vi "MGCC_Version2_MGCC_FntStaMach_Visualization_OpalRT_HTBtwoBatt.vi"() -> ()   [LabVIEW 2016]
doc: "-----------------------------------------------------------------------------------------------------------------------\nCopyright <2019> <The University of Tennessee at Knoxville and the University of Tennessee Research Foundation>\nThis software is released under BSD-3 \nhttps://opensource.org/licenses/BSD-3-Clause \nAdditional license options available at https://utrf.tennessee.edu/industry/sample-agreements/\n-----------------------------------------------------------------------------------------------------------------------"
uses:
  Islanded Control/MGCC_IsdCon_global1.vi
  Resynchronization/MGCC_Resync_global.vi
  Model Management/Global_MdlMgmt.vi
  Communication/Global communication output.vi
  MGCC_FntStaMach_PV_Mode.vi
  PV Forecasting/Sub-VIs/f_MGCC_PVFcst_ActualPV.vi
  Communication/Global communication.vi
  Energy Management/Sub-VIs/f_MGCC_EnergyMgmt_CostSavings.vi
  Energy Management/Sub-VIs/Battery Dispatch.vi
  MGCC_FntStaMach_gobal.vi
  Abnormal Fault State Control/Sub_VIs/Fault_Abnormal_state.vi
  PV Forecasting/Lib/MGCC_PVFcst_dataIO.lvlib
  Energy Management/Lib/MGCC_EnergyMgmt_dataIO.lvlib
panel:
  out "Working state":string
  out "Red":bool
  out "Orange":bool
  out "Yellow":bool
  out "Green":bool
  out "MG Error State":errorcluster
  out "Battery Dispatch GC":dbl[](graph)
  out "Savings":dbl
  out "Communication":bool
  out "PV Forecast":dynamicdata(graph)
  out "APF 8":dbl format="%#.4f"
  out "APF 7":dbl format="%#.4f"
  out "APF 6":dbl format="%#.4f"
  out "APF 5":dbl format="%#.4f"
  out "APF 4":dbl format="%#.4f"
  out "APF 3":dbl format="%#.4f"
  out "APF 2":dbl format="%#.4f"
  out "APF 1":dbl format="%#.4f"
  out "?":bool
  out "?":bool
  out "?":bool
  in  "Load Mode":bool
  in  "?":dbl(slide) scale=0.0..2.0
  in  "PV Mode":bool
  out "Communication":bool
  out "Active power control":bool
  out "Reactive power control":bool
  out "Output":dbl format="%#_4f"
  out "Communication":bool
  out "Resynchronization":bool
  out "Active power control":bool
  out "Reactive power control":bool
  out "SOC 3":dbl format="%#_4f"
  out "Output":dbl format="%#_4f"
  out "Communication":bool
  out "Resynchronization":bool
  out "Active power control":bool
  out "Reactive power control":bool
  out "SOC":dbl format="%#_4f"
  out "Output":dbl format="%#_4f"
  out "I 8":dbl format="%#.4f"
  out "I 7":dbl format="%#.4f"
  out "I 6":dbl format="%#.4f"
  out "I 5":dbl format="%#.4f"
  out "I 4":dbl format="%#.4f"
  out "I 3":dbl format="%#.4f"
  out "I 2":dbl format="%#.4f"
  out "I 1":dbl format="%#.4f"
  out "Current State":string
  out "Model Mgmt.":bool
  out "PV Forecasting":bool
  out "Load Forecasting":bool
  out "PQ Balance":bool
  out "Black Start":bool
  out "Data Logging":bool
  out "State Estimation":bool
  out "Energy Mgmt.":bool
  out "L6":cluster{dbl[], dbl[]}(graph)
  out "L7":cluster{dbl[], dbl[]}(graph)
  out "L8":cluster{dbl[], dbl[]}(graph)
  out "B10":cluster{dbl[], dbl[]}(graph)
  out "PV":cluster{dbl[], dbl[]}(graph)
  out "L11":cluster{dbl[], dbl[]}(graph)
  out "L5":cluster{dbl[], dbl[]}(graph)
  out "G4":cluster{dbl[], dbl[]}(graph)
  out "B12":cluster{dbl[], dbl[]}(graph)
  out "L3":cluster{dbl[], dbl[]}(graph)
  out "L2":cluster{dbl[], dbl[]}(graph)
  out "G1":cluster{dbl[], dbl[]}(graph)
  in  "Stop":bool
  in  "RESET":bool
  in  "G2":bool
  in  "G1":bool
  in  "Ready for STD":bool
  in  "Recon cmd":bool
  in  "BKS cmd":bool
  in  "island cmd":bool
  out "Sources Power":T1(graph)
  in  "Power Tabs":T2(tab)
  out "Loads Power 2":dbl(graph)
  out "Loads Power 3":dbl(graph)
  out "Loads Power 5":dbl(graph)
  out "Loads Power 6":dbl(graph)
  out "Loads Power 7":dbl(graph)
  out "Loads Power 8":dbl(graph)
  out "Loads Power 11":dbl(graph)
  in  "Voltage Tabs":T2(tab)
  out "Voltage 2":dbl(graph)
  out "Voltage 3":dbl(graph)
  out "Voltage 5":dbl(graph)
  out "Voltage 6":dbl(graph)
  out "Voltage 7":dbl(graph)
  out "Voltage 8":dbl(graph)
  out "Voltage 11":dbl(graph)
  out "L6":bool
  out "L7":bool
  out "L8":bool
  out "B1":bool
  out "Bess1 Slider":dbl(slide) scale=0.0..1.0
  out "PV":bool
  out "L11":bool
  out "W9":bool
  out "I6":bool
  out "W5":bool
  out "I7":bool
  out "W6":bool
  out "I8":bool
  out "W7":bool
  out "I5":bool
  out "I4":bool
  out "W4":bool
  out "W3":bool
  out "I3":bool
  out "W8":bool
  out "I2":bool
  out "W2":bool
  out "I1":bool
  out "W1":bool
  out "L5":bool
  out "G4":bool
  out "B12":bool
  out "Bess2 Slider":dbl(slide) scale=0.0..1.0
  out "L3":bool
  out "L2":bool
  out "G1":bool
  # "Controller for Microgrid with Dynamic Boundary"
  # "Central Controller"
  # "BESS 12 Local Controller"
  # "BESS12"
  # "G4"
  # "L5"
  # "G1"
  # "L2"
  # "L3"
  # "Load profile \ncontrol"
  # "-Profile"
  # "-Manual"
  # "BESS10"
  # "L8"
  # "L6"
  # "PV9"
  # "L11"
  # "L7"
  # "PV9 Local Controller"
  # "BESS 10 Local Controller"
  # "-Profile"
  # "-Manual"
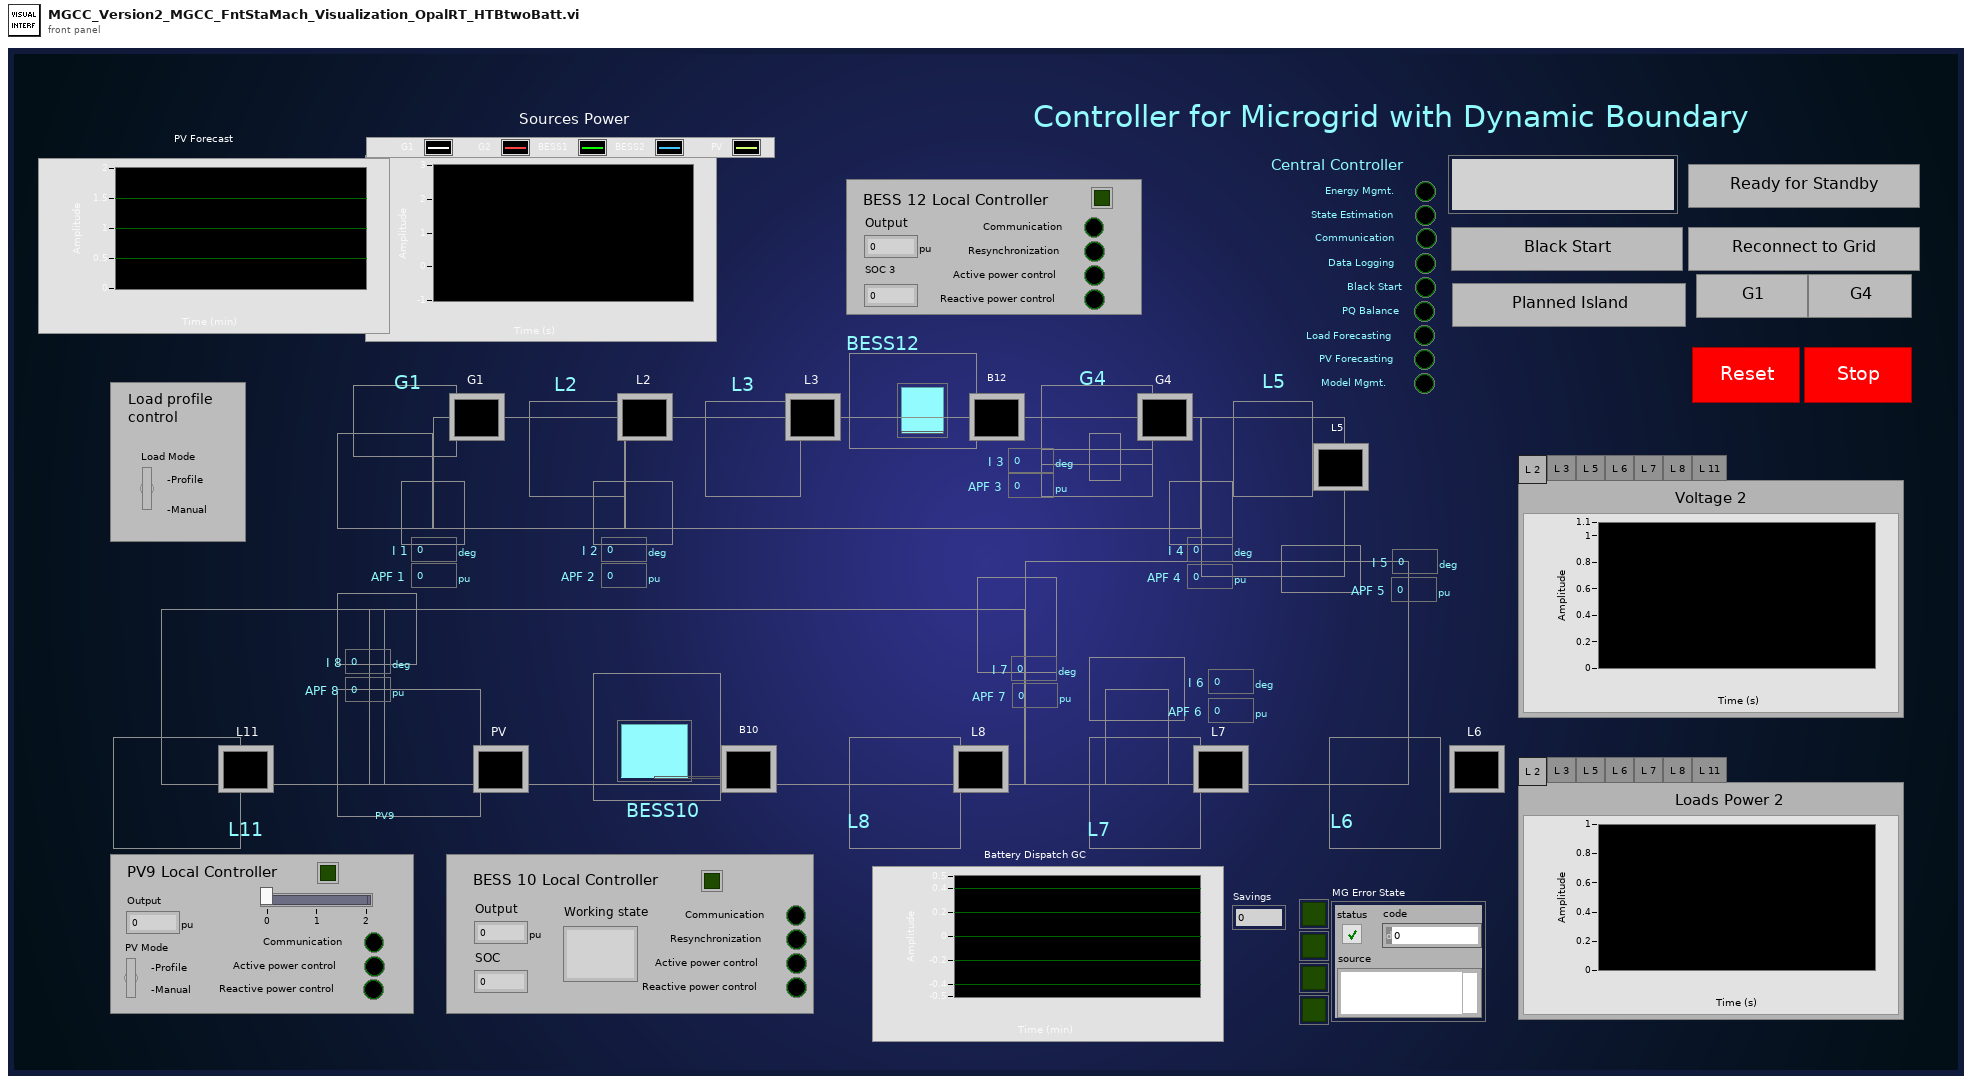
[diagram p1: front panel]
types:
  T1 = cluster{"Double":dbl, "Double":dbl, "Double":dbl, "Double":dbl, "Double":dbl}
  T2 = enum32{"L 2", "L 3", "L 5", "L 6", "L 7", "L 8", "L 11"}
  T3 = cluster{"Numeric":dbl, "Numeric":dbl, "Numeric":dbl, "Numeric":dbl}
  T4 = cluster{"Numeric":dbl, dbl, "Numeric":dbl, "Numeric":dbl, "Numeric":dbl}
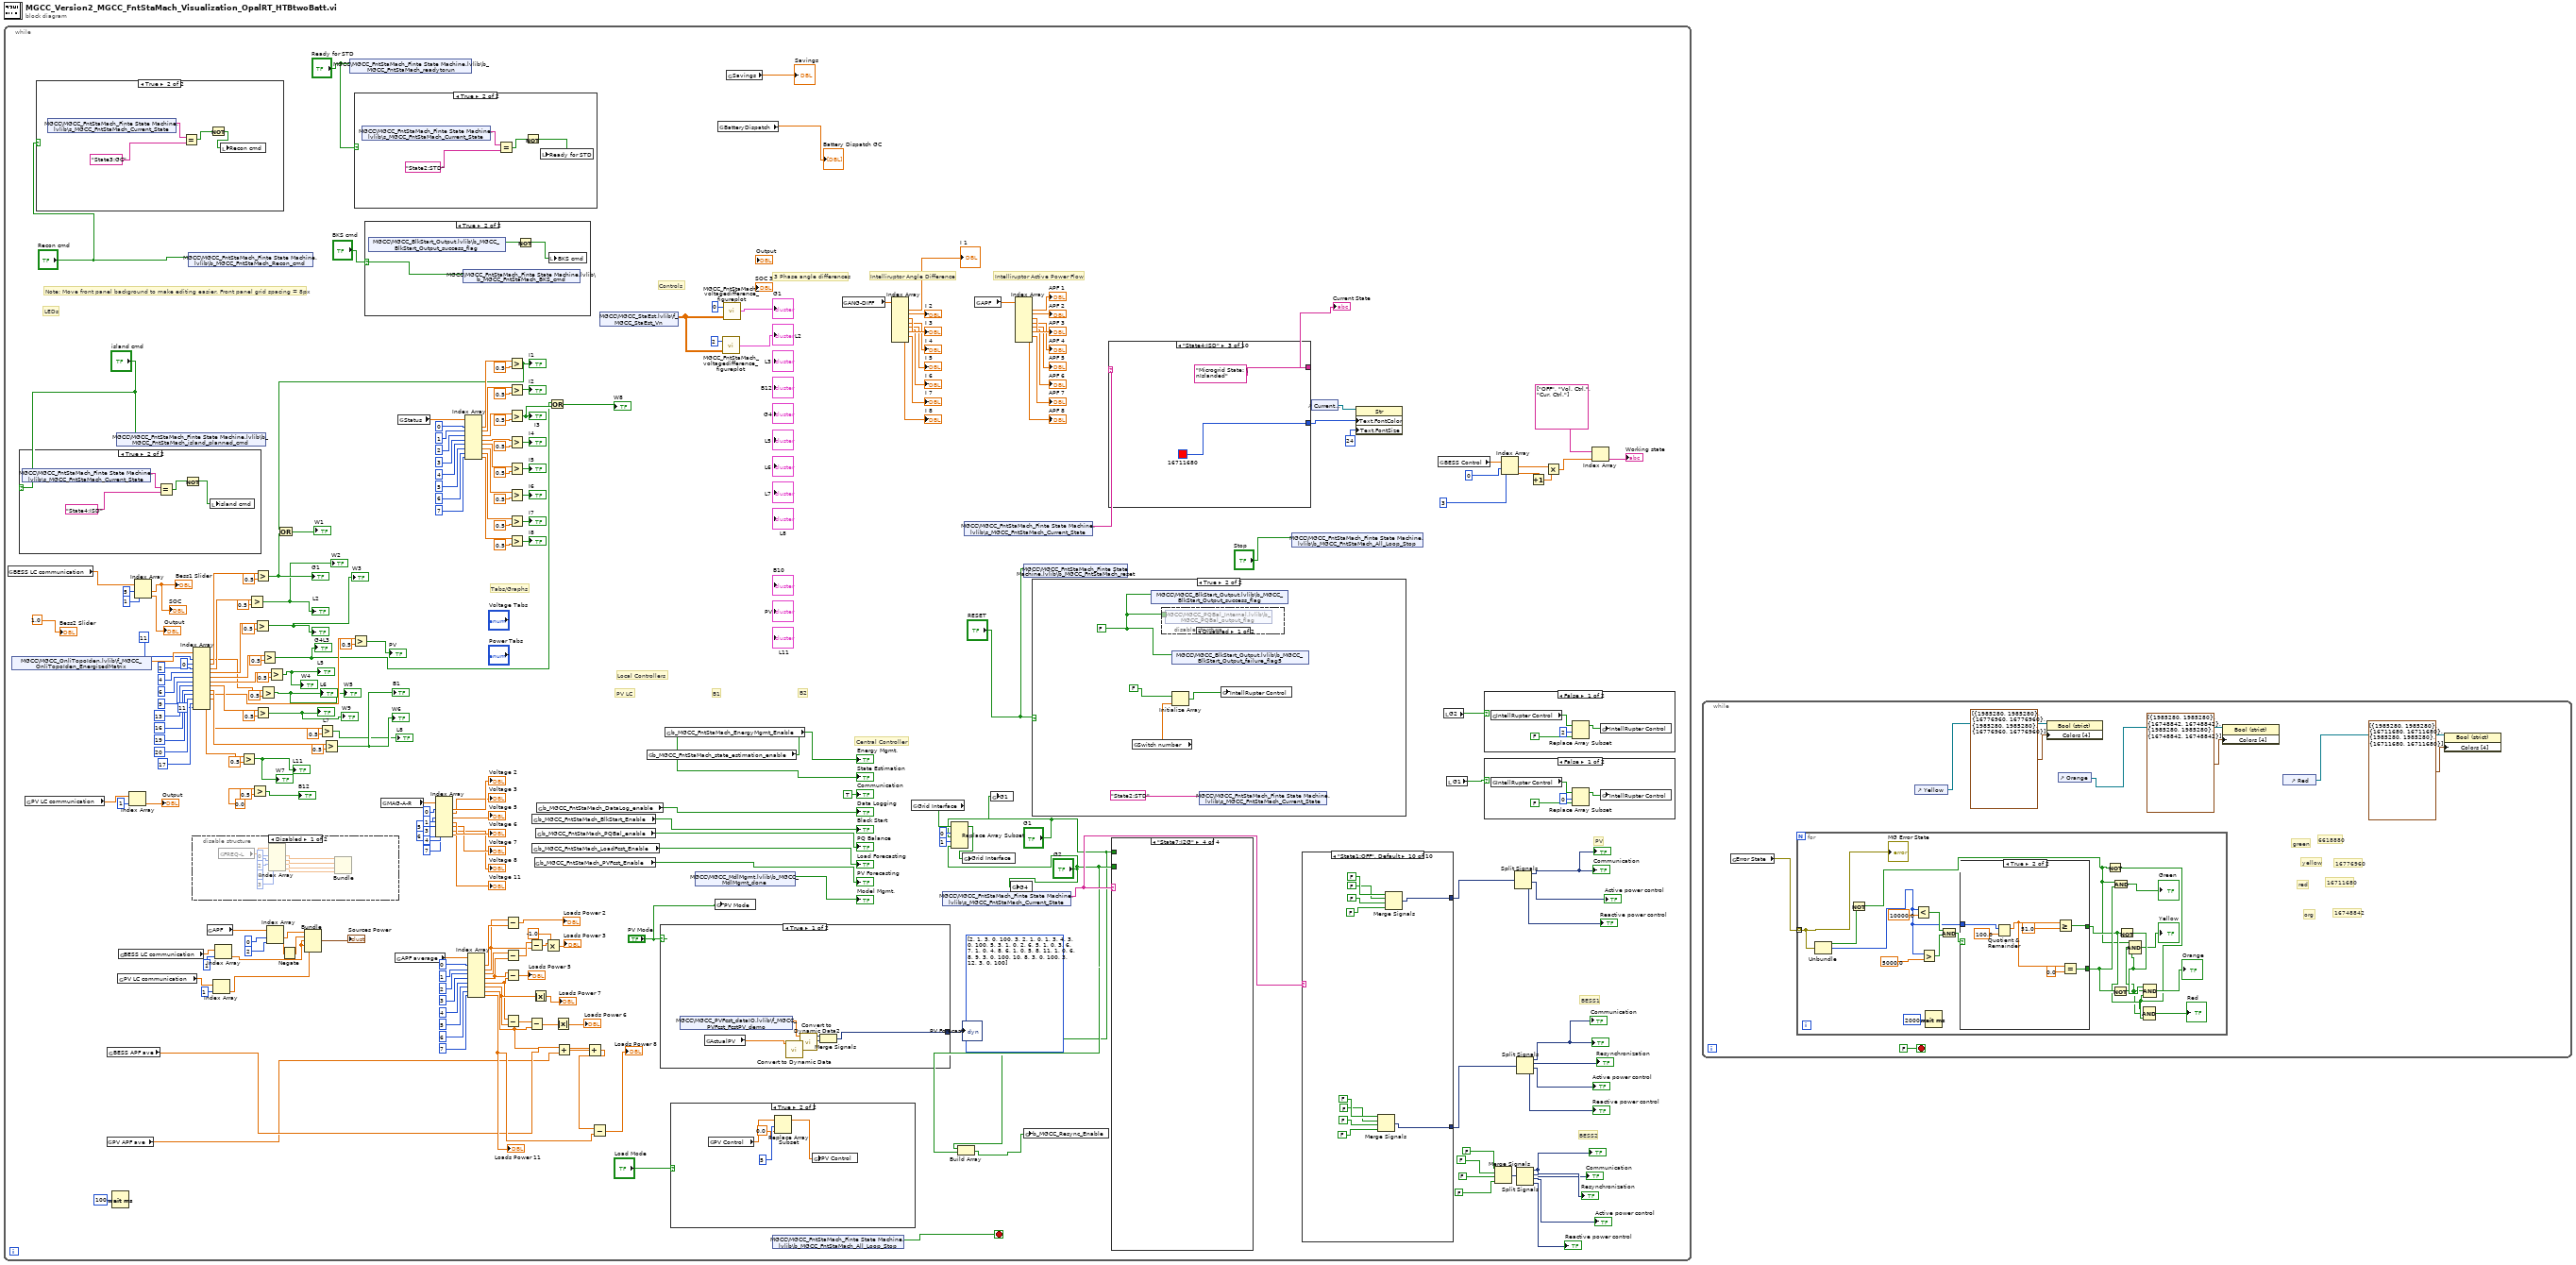
[diagram p0: block diagram]
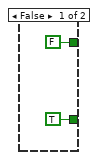
[diagram p2: hidden frame]
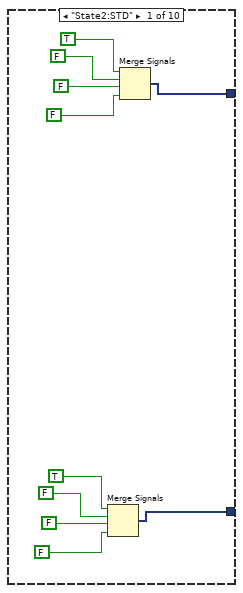
[diagram p8: hidden frame]
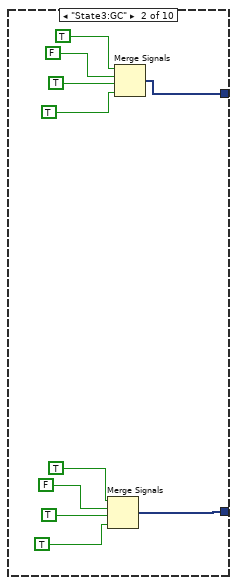
[diagram p9: hidden frame]
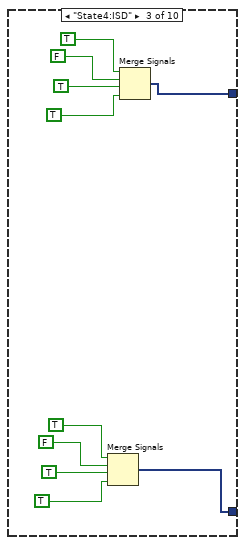
[diagram p10: hidden frame]
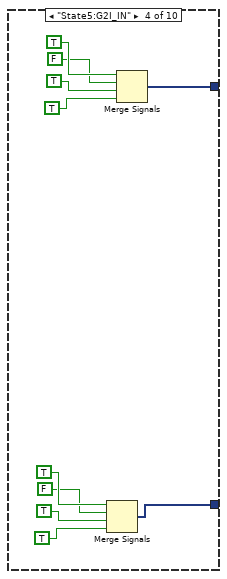
[diagram p11: hidden frame]
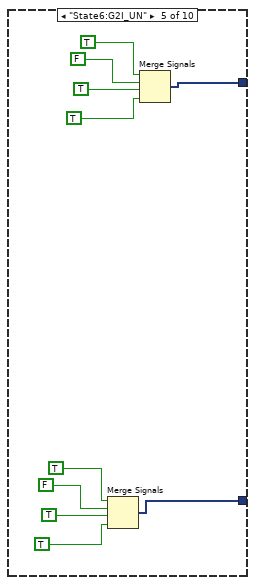
[diagram p12: hidden frame]
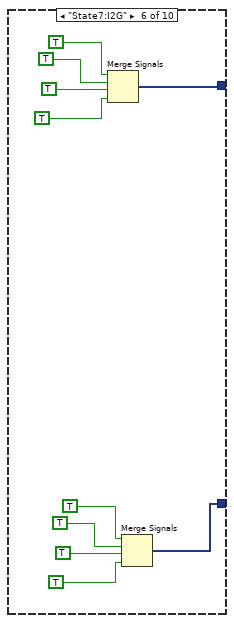
[diagram p13: hidden frame]
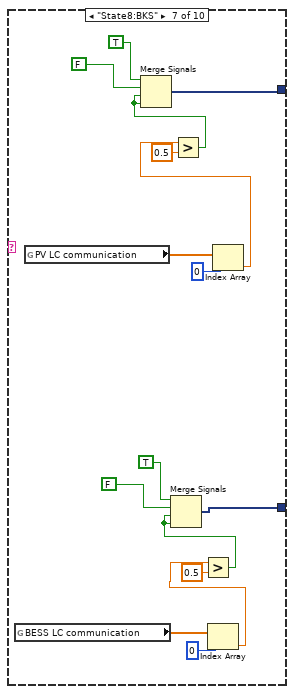
[diagram p14: hidden frame]
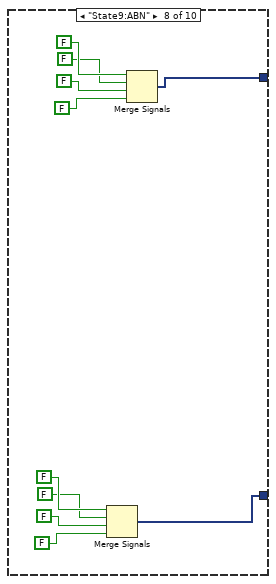
[diagram p15: hidden frame]
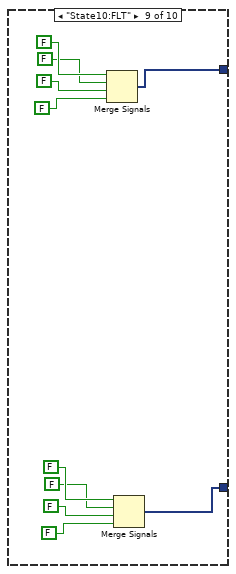
[diagram p16: hidden frame]
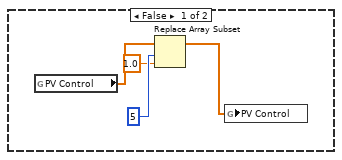
[diagram p18: hidden frame]
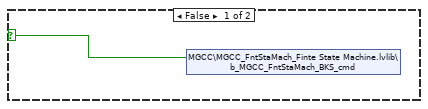
[diagram p19: hidden frame]
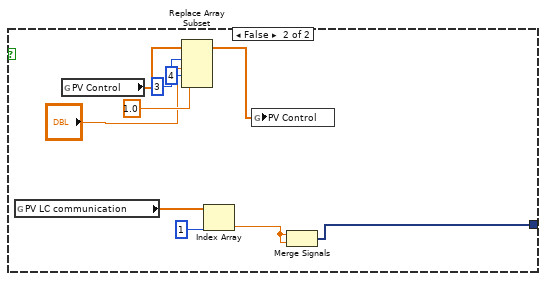
[diagram p20: hidden frame]
diagram:
  n1 = while {
    stop <- w239 stop-if-true
    (unwired) i32[][] [[2, 1, 3, 0, 100], [3, 2, 1, 0, 1], [3, 4, 3, 0, 100], [5, 3, 1, 0, 2], [6, 5, 1, 0, 3], [6, 7, 1, 0, 4], [8, 6, 1, 0, 5], [8, 11, 1, 0, 6], [8, 9, 3, 0, 100], [10, 8, 3, 0, 100], [3, 12, 3, 0, 100]]
    # "Intelliruptor Active Power Flow"
    # "BESS2"
    # "BESS1"
    # "PV"
    # "Note: Move front panel background to make editing easier. Front panel grid spacing = 8px"
    # "Intelliruptor Angle Difference"
    # "B1"
    # "Central Controller"
    # "Local Controllers"
    # "B2"
    # "PV LC"
    # "3 Phase angle differences"
    # "Controls"
    # "Tabs/Graphs"
    # "LEDs"
    n2 = global read "Global communication.vi" "BESS LC communication"() -> (w49:dbl[])
    n3 = shared-variable "MGCC\\MGCC_OnliTopoIden.lvlib\\f_MGCC_OnliTopoIden_EnergizedMatrix"() -> (w238:dbl[])  [unwired: 1 in, 1 out]
    n4 = case shown="True" "island cmd" {
      frame False {
      }
      frame True {
        n5 = shared-variable "MGCC\\MGCC_FntStaMach_Finte State Machine.lvlib\\s_MGCC_FntStaMach_Current_State"() -> (w252:string)  [unwired: 1 in, 1 out]
        n6 = Equal?(x=w252, y="State4:ISD") -> (x = y?=w250:bool)
        n7 = Not(x=w250) -> (.not. x?=w249:bool)
        n8 = local write "island cmd"(w249) -> ()
      }
    }
    n9 = global read "Global communication.vi" "PV LC communication"() -> (w43:dbl[])
    n10 = case shown="True" "Recon cmd" {
      frame False {
      }
      frame True {
        n11 = shared-variable "MGCC\\MGCC_FntStaMach_Finte State Machine.lvlib\\s_MGCC_FntStaMach_Current_State"() -> (w256:string)  [unwired: 1 in, 1 out]
        n12 = Equal?(x=w256, y="State3:GC") -> (x = y?=w254:bool)
        n13 = Not(x=w254) -> (.not. x?=w253:bool)
        n14 = local write "Recon cmd"(w253) -> ()
      }
    }
    n15 = global read "Global communication.vi" "PV APF ave"() -> (w99:dbl)
    n16 = global read "Global communication.vi" "BESS APF ave"() -> (w100:dbl)
    n17 = Wait (ms)(milliseconds to wait=u32 100) -> ()  [unwired: 1 out]
    n18 = shared-variable "MGCC\\MGCC_FntStaMach_Finte State Machine.lvlib\\b_MGCC_FntStaMach_island_planned_cmd"("island cmd") -> ()  [unwired: 1 in, 1 out]
    n19 = global read "Global communication.vi" "PV LC communication"() -> (w143:dbl[])
    n20 = global read "Global communication.vi" "BESS LC communication"() -> (w144:dbl[])
    n21 = Index Array(array=w43, index=1) -> (element=→"Output":dbl)
    n22 = Index Array(array=w49, index #1=5 ("index"), index #2=1 ("index")) -> (element #1=→"Bess1 Slider" →"SOC":dbl, element #2=→"Output":dbl)
    n23 = shared-variable "MGCC\\MGCC_FntStaMach_Finte State Machine.lvlib\\b_MGCC_FntStaMach_Recon_cmd"("Recon cmd") -> ()  [unwired: 1 in, 1 out]
    n24 = disable-structure shown="Disabled" {
      frame Disabled {
        n25 = global read "Global communication.vi" "FREQ-L"() -> (w376:dbl[])
        n26 = Index Array(array=w376, index #1=0 ("index"), index #2=2 ("index"), index #3=6 ("index"), index #4=3 ("index")) -> (element #1=w372:dbl, element #2=w371:dbl, element #3=w370:dbl, element #4=w368:dbl)
        n27 = Bundle("Numeric"=w372, "Numeric"=w371, "Numeric"=w370, "Numeric"=w368) -> (w367:T3)  [unwired: 1 in]
      }
      frame Enabled {
      }
    }
    n28 = Index Array(array=w238, index #1=11 ("index"), index #2=0 ("index"), index #3=2 ("index"), index #4=4 ("index"), index #5=6 ("index"), index #6=9 ("index"), index #7=13 ("index"), index #8=16 ("index"), index #9=19 ("index"), index #10=20 ("index"), index #11=17 ("index"), index #12=11 ("index")) -> (element #1=w209:dbl, element #2=w220:dbl, element #3=w218:dbl, element #4=w216:dbl, element #5=w213:dbl, element #6=w211:dbl, element #7=w207:dbl, element #8=w223:dbl, element #9=w202:dbl, element #10=w227:dbl, element #11=w205:dbl)  [unwired: 1 out]
    n29 = global read "Global communication.vi" "APF"() -> (w147:dbl[])
    n30 = Index Array(array=w143, index=1) -> (element=w108:dbl)
    n31 = Index Array(array=w144, index=1) -> (element=w103:dbl)
    n32 = Greater?(x=w205, y=0.5) -> (0:→"W7" →"L11":bool)
    n33 = Greater?(x=w218, y=0.5) -> (0:→"L2" →"W2":bool)
    n34 = Greater?(x=0.0, y=0.5) -> (0:→"B12":bool)
    n35 = Greater?(x=w216, y=0.5) -> (0:→"L3" →"W3":bool)
    n36 = Greater?(x=w220, y=0.5) -> (0:w167:bool)
    "G1" <- w167
    n37 = Greater?(x=w207, y=0.5) -> (0:→"W9" →"L7":bool)
    n38 = Greater?(x=w209, y=0.5) -> (0:→"W5" →"L6":bool)
    n39 = Greater?(x=w213, y=0.5) -> (0:w157:bool)
    "G4" <- w157
    n40 = Index Array(array=w147, index #1=0 ("index"), index #2=2 ("index")) -> (element #1=w140:dbl, element #2=w139:dbl)
    n41 = Greater?(x=w211, y=0.5) -> (0:→"L5" →"W4":bool)
    n42 = Negate(x=w139) -> (-x=w41:dbl)
    n43 = Bundle("Numeric"=w140, w41, "Numeric"=w103, "Numeric"=w103, "Numeric"=w108) -> (→"Sources Power":T4)  [unwired: 1 in]
    n44 = Greater?(x=w223, y=0.5) -> (0:→"L8":bool)
    n45 = Greater?(x=w227, y=0.5) -> (0:→"W6" →"B1":bool)
    n46 = shared-variable "MGCC\\MGCC_FntStaMach_Finte State Machine.lvlib\\b_MGCC_FntStaMach_readytorun"("Ready for STD") -> ()  [unwired: 1 in, 1 out]
    n47 = Greater?(x=w202, y=0.5) -> (0:→"PV":bool)
    n48 = case shown="True" "Ready for STD" {
      frame False {
      }
      frame True {
        n49 = shared-variable "MGCC\\MGCC_FntStaMach_Finte State Machine.lvlib\\s_MGCC_FntStaMach_Current_State"() -> (w260:string)  [unwired: 1 in, 1 out]
        n50 = Equal?(x=w260, y="State2:STD") -> (x = y?=w258:bool)
        n51 = Not(x=w258) -> (.not. x?=w257:bool)
        n52 = local write "Ready for STD"(w257) -> ()
      }
    }
    n53 = case shown="True" "BKS cmd" {
      selector: "BKS cmd" -> [w385 w388]
      frame False {
        n54 = shared-variable "MGCC\\MGCC_FntStaMach_Finte State Machine.lvlib\\b_MGCC_FntStaMach_BKS_cmd"(w385) -> ()  [unwired: 1 in, 1 out]
      }
      frame True {
        n55 = shared-variable "MGCC\\MGCC_BlkStart_Output.lvlib\\b_MGCC_BlkStart_Output_success_flag"() -> (w386:bool)  [unwired: 1 in, 1 out]
        n56 = shared-variable "MGCC\\MGCC_FntStaMach_Finte State Machine.lvlib\\b_MGCC_FntStaMach_BKS_cmd"(w388) -> ()  [unwired: 1 in, 1 out]
        n57 = Not(x=w386) -> (.not. x?=w387:bool)
        n58 = local write "BKS cmd"(w387) -> ()
      }
    }
    n59 = global read "Global communication.vi" "MAG-A-R"() -> (w138:dbl[])
    n60 = global read "Global communication.vi" "APF average"() -> (w123:dbl[])
    n61 = global read "Global communication.vi" "Status"() -> (w198:dbl[])
    n62 = Index Array(array=w138, index #1=0 ("index"), index #2=1 ("index"), index #3=3 ("index"), index #4=4 ("index"), index #5=5 ("index"), index #6=6 ("index"), index #7=7 ("index")) -> (element #1=→"Voltage 2":dbl, element #2=→"Voltage 3":dbl, element #3=→"Voltage 5":dbl, element #4=→"Voltage 6":dbl, element #5=→"Voltage 7":dbl, element #6=→"Voltage 8":dbl, element #7=→"Voltage 11":dbl)
    n63 = Index Array(array=w198, index #1=0 ("index"), index #2=1 ("index"), index #3=2 ("index"), index #4=3 ("index"), index #5=4 ("index"), index #6=5 ("index"), index #7=6 ("index"), index #8=7 ("index")) -> (element #1=w181:dbl, element #2=w180:dbl, element #3=w179:dbl, element #4=w169:dbl, element #5=w170:dbl, element #6=w171:dbl, element #7=w172:dbl, element #8=w173:dbl)
    n64 = Index Array(array=w123, index #1=0 ("index"), index #2=1 ("index"), index #3=2 ("index"), index #4=3 ("index"), index #5=4 ("index"), index #6=5 ("index"), index #7=6 ("index"), index #8=7 ("index")) -> (element #1=w114:dbl, element #2=w111:dbl, element #3=w113:dbl, element #4=w35:dbl, element #5=w34:dbl, element #6=w106:dbl, element #7=w87:dbl, element #8=w102:dbl)
    "Loads Power 11" <- w102
    n65 = Subtract(x=w111, y=w114) -> (x-y=→"Loads Power 2":dbl)
    n66 = Subtract(x=w113, y=w35) -> (x-y=w112:dbl)
    n67 = Subtract(x=w35, y=w34) -> (x-y=→"Loads Power 5":dbl)
    n68 = Subtract(x=w34, y=w106) -> (x-y=w109:dbl)
    n69 = Greater?(x=w181, y=0.5) -> (0:w166:bool)
    "I1" <- w166
    n70 = Or(x=w166, y=w167) -> (x .or. y?=→"W1":bool)
    n71 = Greater?(x=w180, y=0.5) -> (0:→"I2":bool)
    n72 = Greater?(x=w179, y=0.5) -> (0:w158:bool)
    "I3" <- w158
    n73 = Greater?(x=w169, y=0.5) -> (0:→"I4":bool)
    n74 = Greater?(x=w170, y=0.5) -> (0:→"I5":bool)
    n75 = Greater?(x=w171, y=0.5) -> (0:→"I6":bool)
    n76 = Greater?(x=w172, y=0.5) -> (0:→"I7":bool)
    n77 = Greater?(x=w173, y=0.5) -> (0:→"I8":bool)
    n78 = Subtract(x=w112, y=w111) -> (x-y=w38:dbl)
    n79 = Subtract(x=w109, y=w87) -> (x-y=w105:dbl)
    n80 = global read "MGCC_FntStaMach_gobal.vi" "b_MGCC_FntStaMach_BlkStart_Enable"() -> (→"Black Start":bool)
    n81 = global read "MGCC_FntStaMach_gobal.vi" "b_MGCC_FntStaMach_LoadFcst_Enable"() -> (→"Load Forecasting":bool)
    n82 = Absolute Value(x=w106) -> (abs(x)=→"Loads Power 7":dbl)
    n83 = global read "MGCC_FntStaMach_gobal.vi" "b_MGCC_FntStaMach_PVFcst_Enable"() -> (→"PV Forecasting":bool)
    n84 = global read "MGCC_FntStaMach_gobal.vi" "b_MGCC_FntStaMach_PQBal_enable"() -> (→"PQ Balance":bool)
    n85 = global read "MGCC_FntStaMach_gobal.vi" "b_MGCC_FntStaMach_DataLog_enable"() -> (→"Data Logging":bool)
    n86 = Multiply(x=w38, y=-1.0) -> (x*y=→"Loads Power 3":dbl)
    n87 = Or(x=w157, y=w158) -> (x .or. y?=→"W8":bool)
    n88 = Absolute Value(x=w105) -> (abs(x)=→"Loads Power 6":dbl)
    n89 = Add(x=w100, y=w99) -> (x+y=w88:dbl)
    n90 = Add(x=w87, y=w88) -> (x+y=w86:dbl)
    n91 = Subtract(x=w86, y=w102) -> (x-y=→"Loads Power 8":dbl)
    n92 = shared-variable "MGCC\\MGCC_StaEst.lvlib\\f_MGCC_StaEst_Vn"() -> (w21:dbl[][])  [unwired: 1 in, 1 out]
    n93 = global read "MGCC_FntStaMach_gobal.vi" "b_MGCC_FntStaMach_state_estimation_enable"() -> (→"State Estimation":bool)
    n94 = case shown="True" "PV Mode" {
      tunnel: [w392 w395] -> w55
      frame True {
        n95 = shared-variable "MGCC\\MGCC_PVFcst_dataIO.lvlib\\f_MGCC_PVFcst_FcstPV_demo"() -> (w391:dbl[])  [unwired: 1 in, 1 out]
        n96 = global read "f_MGCC_PVFcst_ActualPV.vi" "ActualPV"() -> (w389:dbl[])
        n97 = call "Convert to Dynamic Data"("Array"=w389) -> ("Dynamic Data Type"=w393:dynamicdata)  [unwired: 3 in]
        n98 = call "Convert to Dynamic Data2"("Array"=w391) -> ("Dynamic Data Type"=w390:dynamicdata)  [unwired: 3 in]
        n99 = Merge Signals(w390, w393) -> (w392:dynamicdata)
      }
      frame False {
        n100 = global read "Global communication.vi" "PV LC communication"() -> (w397:dbl[])
        n101 = global read "Global communication output.vi" "PV Control"() -> (w401:dbl[])
        n102 = Replace Array Subset(array=w401, new element #1="?", index #1=3 ("index"), new element #2=1.0 ("new element/subarray"), index #2=4 ("index")) -> (w402:dbl[])
        n103 = Index Array(array=w397, index=1) -> (element=w394:dbl)
        n104 = global write "Global communication output.vi" "PV Control"(w402) -> ()
        n105 = Merge Signals(w394, w394) -> (w395:dynamicdata)
      }
    }
    "PV Forecast" <- w55
    n106 = global read "MGCC_FntStaMach_gobal.vi" "b_MGCC_FntStaMach_EnergyMgmt_Enable"() -> (→"Energy Mgmt.":bool)
    n107 = case shown="True" "Load Mode" {
      frame False {
        n108 = global read "Global communication output.vi" "PV Control"() -> (w379:dbl[])
        n109 = Replace Array Subset(array=w379, new element=1.0 ("new element/subarray"), index=5) -> (w380:dbl[])
        n110 = global write "Global communication output.vi" "PV Control"(w380) -> ()
      }
      frame True {
        n111 = global read "Global communication output.vi" "PV Control"() -> (w383:dbl[])
        n112 = Replace Array Subset(array=w383, new element=0.0 ("new element/subarray"), index=5) -> (w384:dbl[])
        n113 = global write "Global communication output.vi" "PV Control"(w384) -> ()
      }
    }
    n114 = shared-variable "MGCC\\MGCC_MdlMgmt.lvlib\\b_MGCC_MdlMgmt_done"() -> (→"Model Mgmt.":bool)  [unwired: 1 in, 1 out]
    n115 = global write "MGCC_FntStaMach_PV_Mode.vi" "PV Mode"("PV Mode") -> ()
    n116 = global read "Battery Dispatch.vi" "BatteryDispatch"() -> (→"Battery Dispatch GC":dbl[])
    n117 = call "MGCC_FntStaMach_voltagedifference_figureplot.vi"("array"=w21, "index (row)"=2) -> ("output cluster"=→"L2":cluster{dbl[], dbl[]})
    n118 = call "MGCC_FntStaMach_voltagedifference_figureplot.vi"("array"=w21, "index (row)"=0) -> ("output cluster"=→"G1":cluster{dbl[], dbl[]})
    n119 = global read "f_MGCC_EnergyMgmt_CostSavings.vi" "Savings"() -> (→"Savings":dbl)
    n120 = shared-variable "MGCC\\MGCC_FntStaMach_Finte State Machine.lvlib\\b_MGCC_FntStaMach_All_Loop_Stop"() -> (w239:bool)  [unwired: 1 in, 1 out]
    n121 = global read "Global communication.vi" "ANG-DIFF"() -> (w98:dbl[])
    n122 = Index Array(array=w98) -> (element #1=→"I 1":dbl, element #2=→"I 2":dbl, element #3=→"I 3":dbl, element #4=→"I 4":dbl, element #5=→"I 5":dbl, element #6=→"I 6":dbl, element #7=→"I 7":dbl, element #8=→"I 8":dbl)  [unwired: 8 in]
    n123 = global read "MGCC_IsdCon_global1.vi" "Grid Interface"() -> (w31:bool[])
    n124 = shared-variable "MGCC\\MGCC_FntStaMach_Finte State Machine.lvlib\\s_MGCC_FntStaMach_Current_State"() -> (w79:string)  [unwired: 1 in, 1 out]
    n125 = Replace Array Subset(array=w31, new element #1="G1", index #1=0 ("index"), new element #2="G2", index #2=1 ("index")) -> (w30:bool[])
    n126 = Build Array("G1", "G2") -> (w89:bool[])
    n127 = global write "MGCC_IsdCon_global1.vi" "Grid Interface"(w30) -> ()
    n128 = shared-variable "MGCC\\MGCC_FntStaMach_Finte State Machine.lvlib\\s_MGCC_FntStaMach_Current_State"() -> (w155:string)  [unwired: 1 in, 1 out]
    n129 = global read "Global communication.vi" "APF"() -> (w64:dbl[])
    n130 = global write "MGCC_IsdCon_global1.vi" "G1"("G1") -> ()
    n131 = global write "MGCC_IsdCon_global1.vi" "G4"("G2") -> ()
    n132 = Index Array(array=w64) -> (element #1=→"APF 1":dbl, element #2=→"APF 2":dbl, element #3=→"APF 3":dbl, element #4=→"APF 4":dbl, element #5=→"APF 5":dbl, element #6=→"APF 6":dbl, element #7=→"APF 7":dbl, element #8=→"APF 8":dbl)  [unwired: 8 in]
    n133 = shared-variable "MGCC\\MGCC_FntStaMach_Finte State Machine.lvlib\\b_MGCC_FntStaMach_reset"("RESET") -> ()  [unwired: 1 in, 1 out]
    n134 = global write "MGCC_Resync_global.vi" "b_MGCC_Resync_Enable"(w89) -> ()
    n135 = case shown="True" "RESET" {
      frame False {
      }
      frame True {
        w407 = FALSE ("S0102-status-ctrl")
        n136 = global read "Global_MdlMgmt.vi" "Switch number"() -> (w404:dbl)
        n137 = shared-variable "MGCC\\MGCC_BlkStart_Output.lvlib\\b_MGCC_BlkStart_Output_success_flag"(w407) -> ()  [unwired: 1 in, 1 out]
        n138 = disable-structure shown="Disabled" {
          disable-tunnel: w407 -> [w409 _]
          frame Disabled {
            n139 = shared-variable "MGCC\\MGCC_PQBal_Internal.lvlib\\b_MGCC_PQBal_output_flag"(w409) -> ()  [unwired: 1 in, 1 out]
          }
          frame Enabled {
          }
        }
        n140 = shared-variable "MGCC\\MGCC_BlkStart_Output.lvlib\\b_MGCC_BlkStart_Output_failure_flag5"(w407) -> ()  [unwired: 1 in, 1 out]
        n141 = Initialize Array(FALSE, w404) -> (w405:bool[])
        n142 = shared-variable "MGCC\\MGCC_FntStaMach_Finte State Machine.lvlib\\s_MGCC_FntStaMach_Current_State"("State2:STD" ("s_MGCC_FntStaMach_Current_State")) -> ()  [unwired: 1 in, 1 out]
        n143 = global write "Global communication output.vi" "IntellRupter Control"(w405) -> ()
      }
    }
    n144 = case shown="\"State4:ISD\"" w155 {
      tunnel: ["Microgrid State: \nOutage" "Microgrid State: \nGrid Connected" "Microgrid State: \nIslanded" "Microgrid State: \nGrid Connected" "Microgrid State: \nGrid Connected" "Microgrid State: \nIslanded" "Microgrid State: \nIslanded" "Current State:\nAbnormal" "Current State:\nFault" "Microgrid State: \nOutage"] -> w153
      tunnel: [u32 16748842 u32 1985280 u32 16711680 u32 1985280 u32 1985280 u32 16711680 u32 16711680 u32 0 u32 0 u32 16748842] -> w152
      frame "State2:STD" {
      }
      frame "State3:GC" {
      }
      frame "State4:ISD" {
      }
      frame "State5:G2I_IN" {
      }
      frame "State6:G2I_UN" {
      }
      frame "State7:I2G" {
      }
      frame "State8:BKS" {
      }
      frame "State9:ABN" {
      }
      frame "State10:FLT" {
      }
      frame "State1:OFF", Default {
      }
    }
    "Current State" <- w153
    n145 = case shown="\"State7:I2G\"" w79 {
      tunnel: "G1" -> [_ _ _ _]
      tunnel: "G2" -> [_ _ _ _]
      frame "State6:G2I_UN" {
      }
      frame "State3:GC" {
        n146 = shared-variable "MGCC\\MGCC_Resync.lvlib\\b_MGCC_Resync_Enable"(bool[] [FALSE, FALSE] ("b_MGCC_Resync_Enable")) -> ()  [unwired: 1 in, 1 out]
      }
      frame "False", Default {
      }
      frame "State7:I2G" {
      }
    }
    n147 = shared-variable "MGCC\\MGCC_FntStaMach_Finte State Machine.lvlib\\b_MGCC_FntStaMach_All_Loop_Stop"("Stop") -> ()  [unwired: 1 in, 1 out]
    n148 = case shown="\"State1:OFF\", Default" w79 {
      tunnel: [w266 w276 w286 w296 w306 w319 w335 w342 w352 w362] -> w78
      tunnel: [w261 w272 w282 w291 w301 w311 w327 w337 w347 w357] -> w74
      frame "State2:STD" {
        n149 = Merge Signals(TRUE ("Resynchronization"), FALSE ("Resynchronization"), FALSE ("Resynchronization"), FALSE ("Resynchronization")) -> (w261:dynamicdata)
        n150 = Merge Signals(TRUE ("Resynchronization"), FALSE ("Resynchronization"), FALSE ("Resynchronization"), FALSE ("Resynchronization")) -> (w266:dynamicdata)
      }
      frame "State3:GC" {
        n151 = Merge Signals(TRUE ("Resynchronization"), FALSE ("Resynchronization"), TRUE ("Resynchronization"), TRUE ("Resynchronization")) -> (w272:dynamicdata)
        n152 = Merge Signals(TRUE ("Resynchronization"), FALSE ("Resynchronization"), TRUE ("Resynchronization"), TRUE ("Resynchronization")) -> (w276:dynamicdata)
      }
      frame "State4:ISD" {
        n153 = Merge Signals(TRUE ("Resynchronization"), FALSE ("Resynchronization"), TRUE ("Resynchronization"), TRUE ("Resynchronization")) -> (w282:dynamicdata)
        n154 = Merge Signals(TRUE ("Resynchronization"), FALSE ("Resynchronization"), TRUE ("Resynchronization"), TRUE ("Resynchronization")) -> (w286:dynamicdata)
      }
      frame "State5:G2I_IN" {
        n155 = Merge Signals(TRUE ("Resynchronization"), FALSE ("Resynchronization"), TRUE ("Resynchronization"), TRUE ("Resynchronization")) -> (w291:dynamicdata)
        n156 = Merge Signals(TRUE ("Resynchronization"), FALSE ("Resynchronization"), TRUE ("Resynchronization"), TRUE ("Resynchronization")) -> (w296:dynamicdata)
      }
      frame "State6:G2I_UN" {
        n157 = Merge Signals(TRUE ("Resynchronization"), FALSE ("Resynchronization"), TRUE ("Resynchronization"), TRUE ("Resynchronization")) -> (w301:dynamicdata)
        n158 = Merge Signals(TRUE ("Resynchronization"), FALSE ("Resynchronization"), TRUE ("Resynchronization"), TRUE ("Resynchronization")) -> (w306:dynamicdata)
      }
      frame "State7:I2G" {
        n159 = Merge Signals(TRUE ("Resynchronization"), TRUE ("Resynchronization"), TRUE ("Resynchronization"), TRUE ("Resynchronization")) -> (w319:dynamicdata)
        n160 = Merge Signals(TRUE ("Resynchronization"), TRUE ("Resynchronization"), TRUE ("Resynchronization"), TRUE ("Resynchronization")) -> (w311:dynamicdata)
      }
      frame "State8:BKS" {
        n161 = global read "Global communication.vi" "BESS LC communication"() -> (w322:dbl[])
        n162 = global read "Global communication.vi" "PV LC communication"() -> (w326:dbl[])
        n163 = Index Array(array=w322, index=0) -> (element=w321:dbl)
        n164 = Greater?(x=w321, y=0.5) -> (0:w329:bool)
        n165 = Merge Signals(TRUE ("Resynchronization"), FALSE ("Resynchronization"), w329, w329) -> (w327:dynamicdata)
        n166 = Index Array(array=w326, index=0) -> (element=w324:dbl)
        n167 = Greater?(x=w324, y=0.5) -> (0:w333:bool)
        n168 = Merge Signals(TRUE ("Resynchronization"), FALSE ("Resynchronization"), w333, w333) -> (w335:dynamicdata)
      }
      frame "State9:ABN" {
        n169 = Merge Signals(FALSE ("Resynchronization"), FALSE ("Resynchronization"), FALSE ("Resynchronization"), FALSE ("Resynchronization")) -> (w337:dynamicdata)
        n170 = Merge Signals(FALSE ("Resynchronization"), FALSE ("Resynchronization"), FALSE ("Resynchronization"), FALSE ("Resynchronization")) -> (w342:dynamicdata)
      }
      frame "State10:FLT" {
        n171 = Merge Signals(FALSE ("Resynchronization"), FALSE ("Resynchronization"), FALSE ("Resynchronization"), FALSE ("Resynchronization")) -> (w352:dynamicdata)
        n172 = Merge Signals(FALSE ("Resynchronization"), FALSE ("Resynchronization"), FALSE ("Resynchronization"), FALSE ("Resynchronization")) -> (w347:dynamicdata)
      }
      frame "State1:OFF", Default {
        n173 = Merge Signals(FALSE ("Resynchronization"), FALSE ("Resynchronization"), FALSE ("Resynchronization"), FALSE ("Resynchronization")) -> (w357:dynamicdata)
        n174 = Merge Signals(FALSE ("Resynchronization"), FALSE ("Resynchronization"), FALSE ("Resynchronization"), FALSE ("Resynchronization")) -> (w362:dynamicdata)
      }
    }
    n175 = control-ref of="Current State"() -> (w154:refnum<vi>)
    n176 = property on="Property Node" class="Str"(reference=w154, "Text.FontColor"=w152, "Text.FontSize"=u32 24 ("Text.Font:Size")) -> ()  [unwired: 1 in, 2 out]
    n177 = global read "Global communication output.vi" "BESS Control"() -> (w17:dbl[])
    n178 = local read "G2"() -> (w32:bool)
    n179 = local read "G1"() -> (w33:bool)
    n180 = case shown="False" w32 {
      frame False {
        n181 = global read "Global communication output.vi" "IntellRupter Control"() -> (w244:bool[])
        n182 = Replace Array Subset(array=w244, new element=FALSE ("new element/subarray"), index=2) -> (w243:bool[])
        n183 = global write "Global communication output.vi" "IntellRupter Control"(w243) -> ()
      }
      frame True {
      }
    }
    n184 = case shown="False" w33 {
      frame False {
        n185 = global read "Global communication output.vi" "IntellRupter Control"() -> (w248:bool[])
        n186 = Replace Array Subset(array=w248, new element=FALSE ("new element/subarray"), index=0) -> (w247:bool[])
        n187 = global write "Global communication output.vi" "IntellRupter Control"(w247) -> ()
      }
      frame True {
      }
    }
    n188 = Merge Signals(FALSE ("Resynchronization"), FALSE ("Resynchronization"), FALSE ("Resynchronization"), FALSE ("Resynchronization")) -> (w65:dynamicdata)
    n189 = Index Array(array=w17, index #1=0 ("index"), index #2=3 ("index")) -> (element #1=w13:dbl, element #2=w14:dbl)
    n190 = Split Signals(w78) -> (→"Communication" →"?":dynamicdata, →"Active power control":dynamicdata, →"Reactive power control":dynamicdata)  [unwired: 4 in, 1 out]
    n191 = Split Signals(w74) -> (→"?" →"Communication":dynamicdata, →"Resynchronization":dynamicdata, →"Active power control":dynamicdata, →"Reactive power control":dynamicdata)  [unwired: 4 in]
    n192 = Split Signals(w65) -> (→"Communication" →"?":dynamicdata, →"Resynchronization":dynamicdata, →"Active power control":dynamicdata, →"Reactive power control":dynamicdata)  [unwired: 4 in]
    n193 = Increment(x=w14) -> (x+1=w12:dbl)
    n194 = Multiply(x=w13, y=w12) -> (x*y=w11:dbl)
    n195 = Index Array(array=string[] ["OFF", "Vol. Ctrl.", "Cur. Ctrl."], index=w11) -> (element=→"Working state":string)
    "Bess2 Slider" <- 1.0 ("Slide 2")
    "Communication" <- TRUE ("Communication")
  }
  n196 = while {
    stop <- FALSE stop-if-true
    # "org"
    # "16748842"
    # "red"
    # "yellow"
    # "green"
    # "16776960"
    # "16711680"
    # "6618880"
    n197 = global read "Fault_Abnormal_state.vi" "Error State"() -> (w437:errorcluster[])
    n198 = for {
      tunnel: w437 -> [w456] mode=indexing
      n199 = Unbundle(w456) -> ("status"=w443:bool, "code"=w450:i32)  [unwired: 1 out]
      n200 = Not(x=w443) -> (.not. x?=w441:bool)
      n201 = Less?(x=w450, y=10000.0) -> (x < y?=w453:bool)
      n202 = Greater?(x=w450, y=5000.0) -> (0:w452:bool)
      n203 = Wait (ms)(milliseconds to wait=u32 2000) -> ()  [unwired: 1 out]
      n204 = And(x=w453, y=w452) -> (x .and. y?=w451:bool)
      n205 = case shown="True" w451 {
        tunnel: [FALSE w464] -> w445
        tunnel: [TRUE w461] -> w448
        tunnel: w450 -> [_ w460]
        frame False {
        }
        frame True {
          n206 = Quotient & Remainder(x=w460, y=100.0) -> (x-y*floor(x/y)=w463:dbl)  [unwired: 1 out]
          n207 = Greater Or Equal?(x=w463, y=51.0) -> (x >= y?=w464:bool)
          n208 = Equal?(x=w463, y=0.0) -> (x = y?=w461:bool)
        }
      }
      n209 = Not(x=w441) -> (.not. x?=w446:bool)
      n210 = Not(x=w448) -> (.not. x?=w440:bool)
      n211 = And(x=w441, y=w448) -> (x .and. y?=→"Green":bool)
      n212 = Not(x=w445) -> (.not. x?=w442:bool)
      n213 = Compound Arithmetic op=AND(w441, w440, w442) -> (→"Yellow":bool)
      n214 = Compound Arithmetic op=AND(w445, w440, w446) -> (→"Red":bool)
      n215 = Compound Arithmetic op=AND(w442, w440, w446) -> (→"Orange":bool)
      "MG Error State" <- w456
    }
    n216 = control-ref of="Yellow"() -> (w436:refnum<vi>)
    n217 = property on="Property Node" class="Bool (strict)"(reference=w436, "Colors [4]"=cluster{u32, u32}[] [{1985280, 1985280}, {16776960, 16776960}, {1985280, 1985280}, {16776960, 16776960}]) -> ()  [unwired: 1 in, 2 out]
    n218 = control-ref of="Orange"() -> (w431:refnum<vi>)
    n219 = property on="Property Node" class="Bool (strict)"(reference=w431, "Colors [4]"=cluster{u32, u32}[] [{1985280, 1985280}, {16748842, 16748842}, {1985280, 1985280}, {16748842, 16748842}]) -> ()  [unwired: 1 in, 2 out]
    n220 = control-ref of="Red"() -> (w432:refnum<vi>)
    n221 = property on="Property Node" class="Bool (strict)"(reference=w432, "Colors [4]"=cluster{u32, u32}[] [{1985280, 1985280}, {16711680, 16711680}, {1985280, 1985280}, {16711680, 16711680}]) -> ()  [unwired: 1 in, 2 out]
  }
